vi "Write isAlive.vi"(8 "error in (no error)":errorcluster, 10 "isAlive":bool, 11 "MotorController in":refnum<class "MotorController.lvclass">) -> (0 "error out":errorcluster, 3 "MotorController out":refnum<class "MotorController.lvclass">)   [LabVIEW 2018, in "MotorController.lvclass"]
uses:
  MotorController.lvclass
  MotorController.lvclass/MotorController.ctl
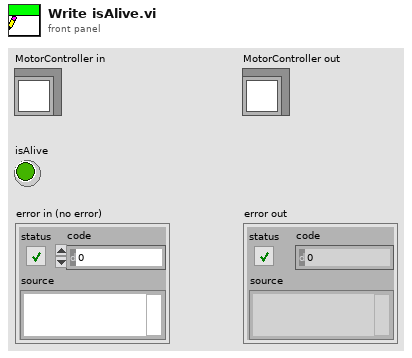
[diagram p1: front panel]
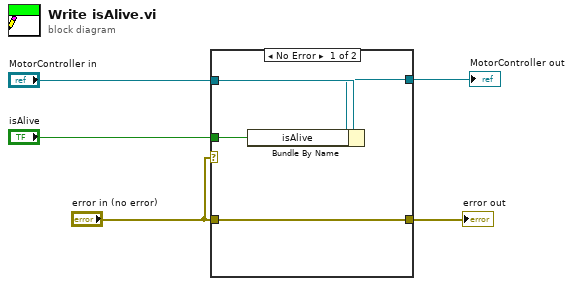
[diagram p0: block diagram]
diagram:
  n1 = case shown="No Error" "error in (no error)" {
    tunnel: "MotorController in" -> [w9 w11]
    tunnel: [w8 w11] -> w4
    tunnel: "isAlive" -> [w7 _]
    tunnel: [w6 w10] -> w2
    tunnel: "error in (no error)" -> [w6 w10]
    frame No Error {
      n2 = Bundle By Name(cluster=w9, "isAlive"=w7) -> (w8:refnum<class "MotorController.lvclass">)
    }
    frame Error {
    }
  }
  "MotorController out" <- w4
  "error out" <- w2
